vi "PLL_Phase and Frequency_PID.vi"() -> ()   [LabVIEW 2019]
doc: "This VI uses a PID controller for both frequency and phase to adjust the frequency and phase of one of the signals to achieve coherency"
uses:
  <vilib>/measure/matone.llb/Extract Single Tone Information 1 Chan.vi
  <vilib>/addons/control/pid/pid.llb/PID (DBL).vi
  <vilib>/measure/NI_MABase.lvlib
  <vilib>/Analysis/NI_AALPro.lvlib
  <vilib>/measure/NI_MAPro.lvlib
  <vilib>/addons/control/pid/NI_PID_pid.lvlib
panel:
  out "Waveform Graph":waveform(dbl)[](graph)=[{"t0"=timestamp(0 s since 1904-01-01), "dt"=0.001, "Y"=array[1000 elements]}, {"t0"=timestamp(0 s since 1904-01-01), "dt"=0.001, "Y"=array[1000 elements]}]
  in  "stop":bool
  in  "Desired Frequency [Hz]":dbl=10.0 format="%_6f"
  # "Overview: This VI uses a PID controller for both frequency and phase to adjust the frequency and phase of one of the signals to achieve coherency\nRequirements: LabVIEW 2012 (or compatible); PID control toolkit 2012 (or compatible)\nInstructions:\n1. Enter the desired signal frequency\n2. Run the VI\n3. Stop Execution"
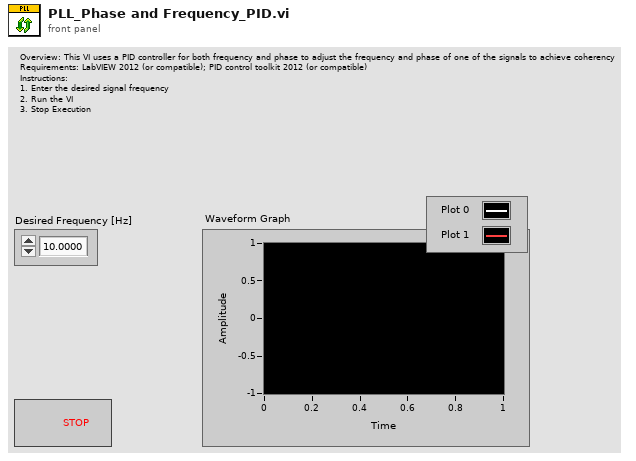
[diagram p1: front panel]
types:
  T1 = cluster{"proportional gain (Kc)":dbl, "integral time (Ti, min)":dbl, "derivative time (Td, min)":dbl}
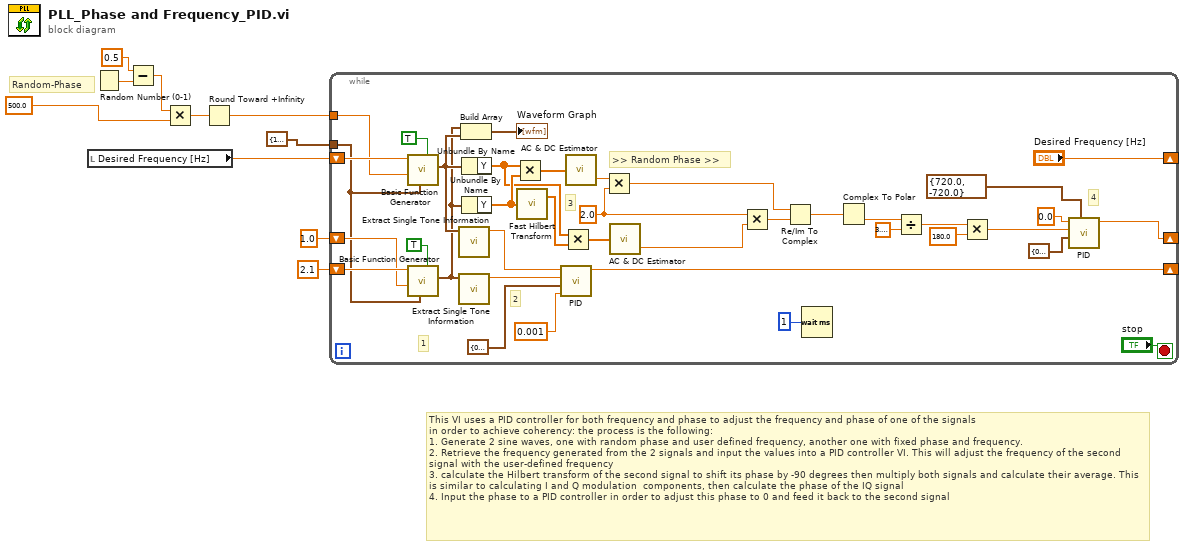
[diagram p0: block diagram]
diagram:
  # "This VI uses a PID controller for both frequency and phase to adjust the frequency and phase of one of the signals \nin order to achieve coherency: the process is the following:\n1. Generate 2 sine waves, one with random phase and user defined frequency, another one with fixed phase and frequency.\n2. Retrieve the frequency generated from the 2 signals and input the values into a PID controller VI. This will adjust the frequency of the second signal with the user-defined frequency\n3. calculate the Hilbert transform of the second signal to shift its phase by -90 degrees then multiply both signals and calculate their average. This is similar to calculating I and Q modulation  components, then calculate the phase of the IQ signal\n4. Input the phase to a PID controller in order to adjust this phase to 0 and feed it back to the second signal"
  # "Random-Phase"
  n1 = local read "Desired Frequency [Hz]"() -> (w1:dbl)
  n2 = Random Number (0-1)() -> (number: 0 to 1=w8:dbl)
  n3 = Subtract(x=0.5, y=w8) -> (x-y=w2:dbl)
  n4 = Multiply(x=w2, y=500.0) -> (x*y=w5:dbl)
  n5 = Round Toward +Infinity(x=w5) -> (ceil(x): smallest int >= x=w4:dbl)
  n6 = while {
    tunnel: cluster{"Fs":dbl, "#s":dbl} {"Fs"=1000.0, "#s"=1000.0} ("sampling info") -> [w11]
    shift-right: [w14] -> _
    shift-left: 1.0 -> [w30]
    tunnel: w4 -> [w17]
    shift-right: [w19] -> _
    shift-left: 2.1 ("f") -> [w44]
    shift-right: ["Desired Frequency [Hz]"] -> _
    shift-left: w1 -> [w23]
    stop <- "stop" stop-if-true
    w28 = 2.0 ("x")
    # "4"
    # "3"
    # "2"
    # "1"
    # ">> Random Phase >>"
    n7 = call <vilib>:"Basic Function Generator.vi"("reset signal"=TRUE, "sampling info"=w11, "phase"=w17, "frequency"=w23) -> ("signal out"=w27:waveform(dbl))  [unwired: 5 in, 2 out]
    n8 = call <vilib>:"Basic Function Generator.vi"("reset signal"=TRUE, "sampling info"=w11, "phase"=w30, "frequency"=w44) -> ("signal out"=w26:waveform(dbl))  [unwired: 5 in, 2 out]
    n9 = call-poly <vilib>:"Extract Single Tone Information.vi"("time signal in"=w27) -> ("detected frequency"=w22:dbl)  [unwired: 5 in, 5 out]
    n10 = call-poly <vilib>:"Extract Single Tone Information.vi"("time signal in"=w26) -> ("detected frequency"=w21:dbl)  [unwired: 5 in, 5 out]
    n11 = Build Array(w26, w27) -> (→"Waveform Graph":waveform(dbl)[])
    n12 = Unbundle By Name(w27) -> ("Y"=w41:dbl[])
    n13 = Unbundle By Name(w26) -> ("Y"=w43:dbl[])
    n14 = Multiply(x=w41, y=w43) -> (x*y=w40:dbl[])
    n15 = call <vilib>:"Fast Hilbert Transform.vi"("X"=w43) -> ("Hilbert{X}"=w42:dbl[])  [unwired: 1 out]
    n16 = call-poly <vilib>:"PID.vi"("dt (s)"=0.001, "PID gains"=T1 {"proportional gain (Kc)"=0.9, "integral time (Ti, min)"=0.0008, "derivative time (Td, min)"=0.0} ("PID_Frequency"), "process variable"=w21, "setpoint"=w22) -> ("output"=w19:dbl)  [unwired: 6 in, 1 out]
    n17 = Multiply(x=w41, y=w42) -> (x*y=w39:dbl[])
    n18 = call <vilib>:"AC & DC Estimator.vi"("Signal (V)"=w40) -> ("DC estimate (V)"=w29:dbl)  [unwired: 1 out]
    n19 = Multiply(x=w29, y=w28) -> (x*y=w32:dbl)
    n20 = call <vilib>:"AC & DC Estimator.vi"("Signal (V)"=w39) -> ("DC estimate (V)"=w38:dbl)  [unwired: 1 out]
    n21 = Multiply(x=w28, y=w38) -> (x*y=w31:dbl)
    n22 = Re/Im To Complex(1:w31, 2:w32) -> (0:w33:cdb)
    n23 = Wait (ms)(milliseconds to wait=u32 1 ("millisecond multiple")) -> ()  [unwired: 1 out]
    n24 = Complex To Polar(r * e^(i*theta)=w33) -> (theta=w34:dbl)  [unwired: 1 out]
    n25 = Divide(x=w34, y=3.141592653589793) -> (x/y=w36:dbl)
    n26 = Multiply(x=w36, y=180.0) -> (x*y=w15:dbl)
    n27 = call-poly <vilib>:"PID.vi"("output range"=cluster{"output high":dbl, "output low":dbl} {"output high"=720.0, "output low"=-720.0}, "PID gains"=T1 {"proportional gain (Kc)"=0.1, "integral time (Ti, min)"=0.0008, "derivative time (Td, min)"=0.0} ("PID_Phase"), "process variable"=w15, "setpoint"=0.0) -> ("output"=w14:dbl)  [unwired: 6 in, 1 out]
  }
